vi "full_add_COUT_(SubVI).vi"(9 "C_in":bool, 10 "B":bool, 11 "A":bool) -> (3 "Boolean":bool)   [LabVIEW 2026]
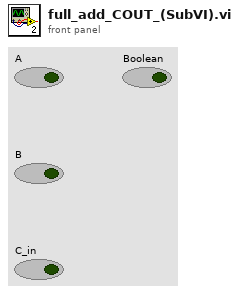
[diagram p1: front panel]
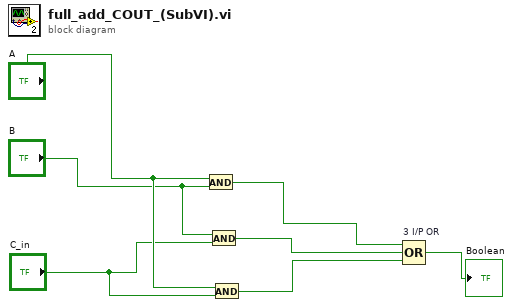
[diagram p0: block diagram]
diagram:
  n1 = And(x="A", y="B") -> (x .and. y?=w4:bool)
  n2 = And(x="B", y="C_in") -> (x .and. y?=w5:bool)
  n3 = And(x="A", y="C_in") -> (x .and. y?=w6:bool)
  n4 = Compound Arithmetic op=OR "3 I/P OR"(w4, w5, w6) -> (→"Boolean":bool)
